vi "OFDM TX - Simulated (No HW).vi"() -> ()   [LabVIEW 2012]
uses:
  <vilib>/addons/Modulation/Analog/controls/Complex Data Waveform.ctl
  <vilib>/addons/Modulation/Digital/General/MT Generate Bits (Galois, PN Order).vi
  <vilib>/addons/Modulation/Digital/General/MT Map Bits to QAM Symbols.vi
  <vilib>/Analysis/2dsp.llb/Inverse Complex FFT.vi
  <vilib>/Analysis/NI_AALPro.lvlib
  <vilib>/addons/Modulation/niDMT.lvlib
  <vilib>/addons/Modulation/niAMT.lvlib
panel:
  out "x*y":cdb[](array[numeric]) format="%#_3g"
  out "Phase":dbl[](graph)
  out "FFT(x)":dbl[](graph)
  in  "Tab Control":T1(tab)=enum."Simulated IQ Impariments"
  in  "IQ rate":dbl=5000000.0 format="%#_6p"
  in  "stop":bool
  out "Outgoing size":i32=1600
  in  "Number of Bits":i32=1250
  in  "error in (no error)":errorcluster
  out "error out":errorcluster
  in  "IQ gain imbalance (dB)":dbl
  in  "frequency offset (Hz)":dbl=250.0
  in  "quadrature skew (deg)":dbl=1.0
  in  "Sample Offset":i32=4
  out "Outgoing Constellation":cdb[](graph)
  # "OFDM Transmitter - Simulated"
  # "Choose offset (0 - 9)"
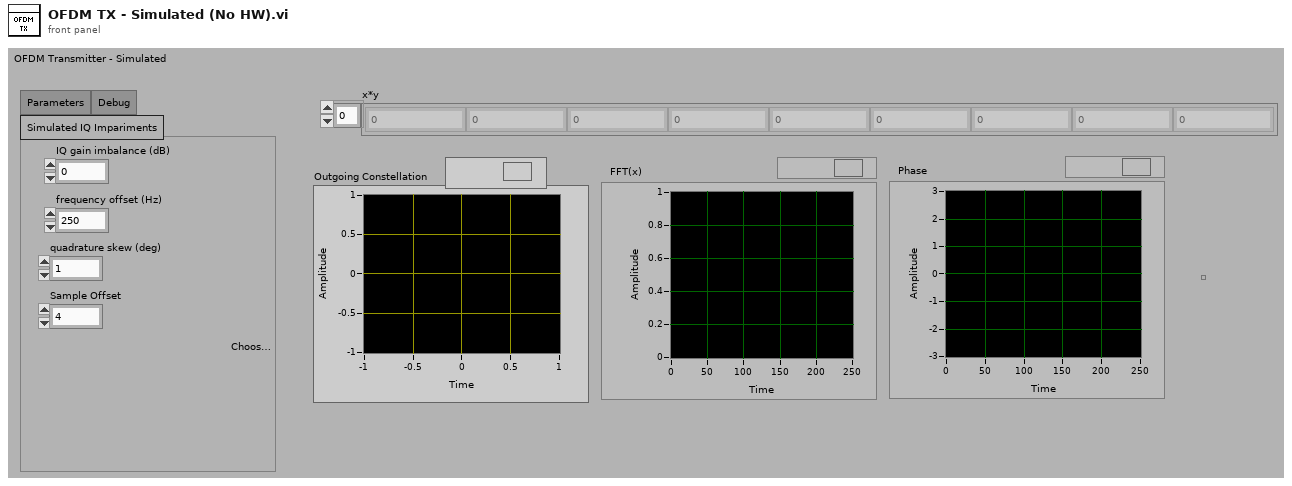
[diagram p1: front panel]
types:
  T1 = enum32{"Parameters", "Debug", "Simulated IQ Impariments"}
  T2 = cluster{"IQ Data":cdb[], "Original Bitstream":i8[]}
  T3 = typedef "niAMT.lvlib/Complex Data Waveform.ctl" = cluster{"t0":dbl, "dt":dbl, "Y":cdb[]}
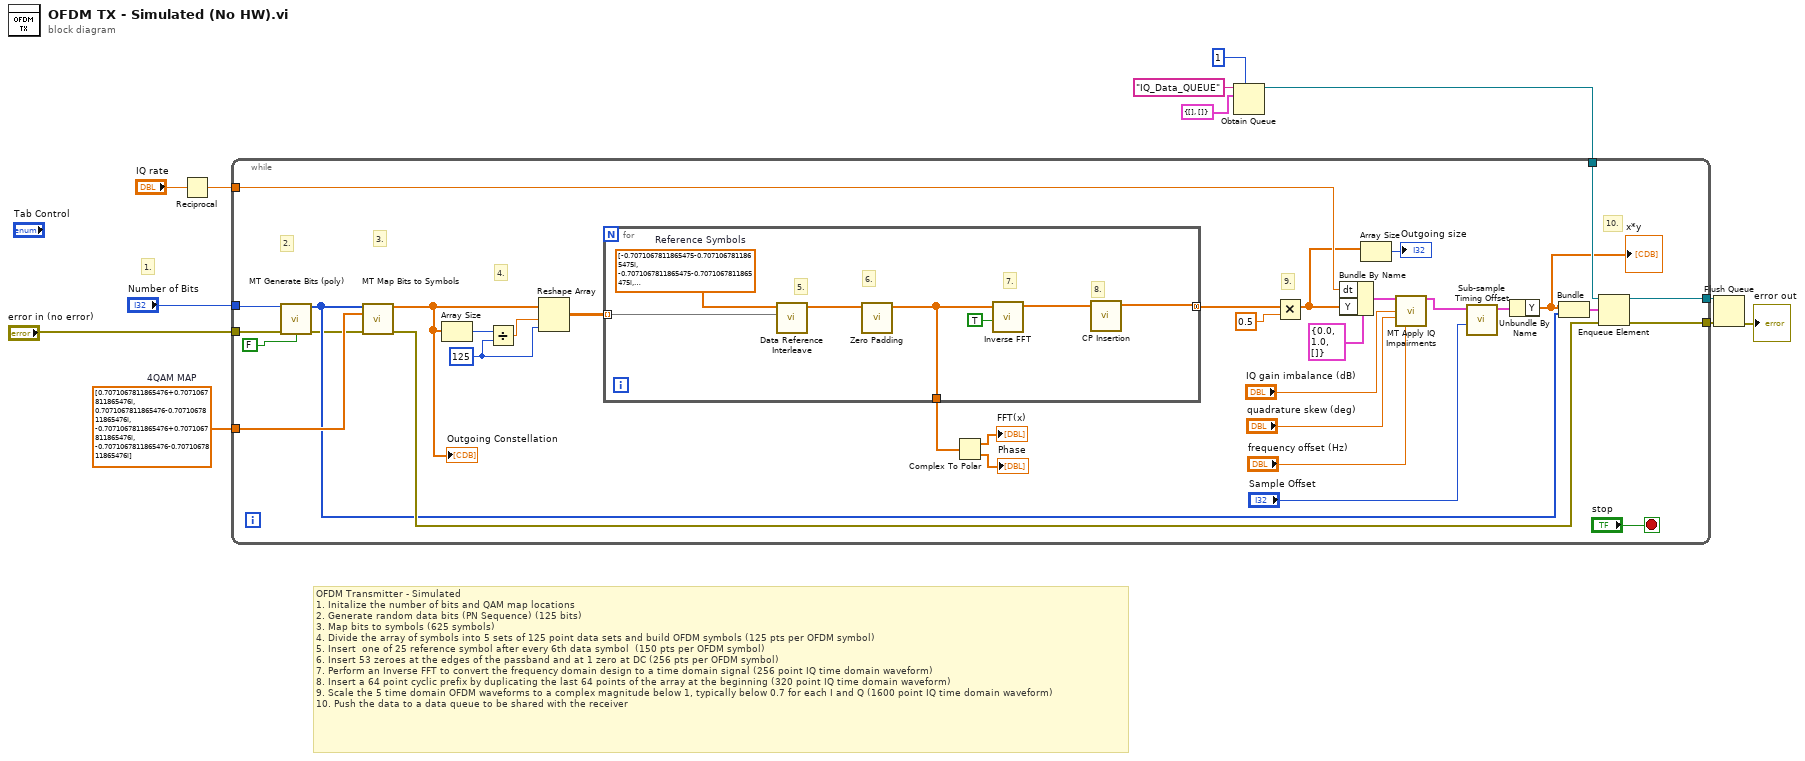
[diagram p0: block diagram]
diagram:
  w12 = cdb[] [0.7071067811865476+0.7071067811865476i, 0.7071067811865476-0.7071067811865476i, -0.7071067811865476+0.7071067811865476i, -0.7071067811865476-0.7071067811865476i]  # 4QAM MAP
  # "1."
  # "OFDM Transmitter - Simulated\n1. Initalize the number of bits and QAM map locations\n2. Generate random data bits (PN Sequence) (125 bits)\n3. Map bits to symbols (625 symbols)\n4. Divide the array of symbols into 5 sets of 125 point data sets and build OFDM symbols (125 pts per OFDM symbol)\n5. Insert  one of 25 reference symbol after every 6th data symbol  (150 pts per OFDM symbol)\n6. Insert 53 zeroes at the edges of the passband and at 1 zero at DC (256 pts per OFDM symbol)\n7. Perform an Inverse FFT to convert the frequency domain design to a time domain signal (256 point IQ time domain waveform)\n8. Insert a 64 point cyclic prefix by duplicating the last 64 points of the array at the beginning (320 point IQ time domain waveform)\n9. Scale the 5 time domain OFDM waveforms to a complex magnitude below 1, typically below 0.7 for each I and Q (1600 point IQ time domain waveform)\n10. Push the data to a data queue to be shared with the receiver"
  n1 = Reciprocal(x="IQ rate") -> (1/x=w3:dbl)
  n2 = Obtain Queue(max queue size (-1, unlimited)=1, name (unnamed)="IQ_Data_QUEUE", element data type=T2 {"IQ Data"=[], "Original Bitstream"=[]} ("output cluster")) -> (queue out=w9:refnum<queue>)  [unwired: 2 in, 2 out]
  n3 = while {
    tunnel: "Number of Bits" -> [w42]
    tunnel: w12 -> [w37]
    tunnel: w9 -> [w31]
    tunnel: [w29] -> w7
    tunnel: [w28] -> w6
    tunnel: w3 -> [w23]
    tunnel: "error in (no error)" -> [w21]
    stop <- "stop" stop-if-true
    w35 = 125 ("y")
    # "10."
    # "9."
    # "4."
    # "3."
    # "2."
    n4 = call-poly <vilib>:"MT Generate Bits (poly).vi"("total bits (128)"=w42, "error in (no error)"=w21, "reset? (T)"=FALSE) -> ("output bit stream"=w15:i8[], "error out"=w13:errorcluster)  [unwired: 10 in, 1 out]
    n5 = call-poly <vilib>:"MT Map Bits to Symbols.vi"("input bit stream"=w15, "symbol map"=w37, "error in (no error)"=w13) -> ("symbols"=w45:cdb[], "error out"=w30:errorcluster)  [unwired: 11 in]
    "Outgoing Constellation" <- w45
    n6 = Array Size(array=w45) -> (size(s)=w44:i32)
    n7 = Divide(x=w44, y=w35) -> (x/y=w43:dbl)
    n8 = Reshape Array(w45, w43, w35) -> (w34:cdb[][])
    n9 = for {
      tunnel: w34 -> [w48] mode=indexing
      tunnel: [w49] -> w32 mode=concatenating
      tunnel: [w51] -> w41
      w47 = cdb[] [-0.7071067811865475-0.7071067811865475i, -0.7071067811865475-0.7071067811865475i, -0.7071067811865475-0.7071067811865475i, 0.7071067811865475-0.7071067811865475i, 0.7071067811865475-0.7071067811865475i, 0.7071067811865475+0.7071067811865475i, 0.7071067811865475-0.7071067811865475i, -0.7071067811865475-0.7071067811865475i, 0.7071067811865475+0.7071067811865475i, -0.7071067811865475+0.7071067811865475i, -0.7071067811865475-0.7071067811865475i, -0.7071067811865475+0.7071067811865475i, -0.7071067811865475+0.7071067811865475i, 0.7071067811865475-0.7071067811865475i, -0.7071067811865475+0.7071067811865475i, -0.7071067811865475+0.7071067811865475i, 0.7071067811865475-0.7071067811865475i, -0.7071067811865475+0.7071067811865475i, -0.7071067811865475-0.7071067811865475i, 0.7071067811865475-0.7071067811865475i, 0.7071067811865475+0.7071067811865475i, -0.7071067811865475-0.7071067811865475i, -0.7071067811865475-0.7071067811865475i, 0.7071067811865475-0.7071067811865475i, -0.7071067811865475-0.7071067811865475i, 0.7071067811865475-0.7071067811865475i, 0.7071067811865475-0.7071067811865475i, 0.7071067811865475+0.7071067811865475i, 0.7071067811865475+0.7071067811865475i, -0.7071067811865475-0.7071067811865475i, -0.7071067811865475+0.7071067811865475i, -0.7071067811865475+0.7071067811865475i, 0.7071067811865475-0.7071067811865475i, -0.7071067811865475-0.7071067811865475i, -0.7071067811865475+0.7071067811865475i, -0.7071067811865475-0.7071067811865475i, -0.7071067811865475+0.7071067811865475i, 0.7071067811865475-0.7071067811865475i, 0.7071067811865475+0.7071067811865475i, 0.7071067811865475+0.7071067811865475i, 0.7071067811865475-0.7071067811865475i, -0.7071067811865475-0.7071067811865475i, -0.7071067811865475+0.7071067811865475i, -0.7071067811865475+0.7071067811865475i, -0.7071067811865475-0.7071067811865475i, -0.7071067811865475-0.7071067811865475i, -0.7071067811865475+0.7071067811865475i, -0.7071067811865475+0.7071067811865475i, -0.7071067811865475+0.7071067811865475i, -0.7071067811865475+0.7071067811865475i]  # Reference Symbols
      # "8."
      # "7."
      # "6."
      # "5."
      n10 = call <userlib>:"Data Reference Interleave.vi"("Data Symbols"=w48, "Reference Symbols"=w47) -> ("Interleaved Output"=w50:cdb[])  [unwired: 9 in]
      n11 = call <userlib>:"Zero Padding.vi"("Array in"=w50) -> ("Array out"=w51:cdb[])  [unwired: 10 in]
      n12 = call-poly <vilib>:"Inverse FFT.vi"("shift?"=TRUE, "FFT {X}"=w51) -> ("X"=w52:cdb[])  [unwired: 8 in, 1 out]
      n13 = call <userlib>:"CP Insertion.vi"("Input"=w52) -> ("Output with CP"=w49:cdb[])  [unwired: 10 in]
    }
    n14 = Complex To Polar(r * e^(i*theta)=w41) -> (r=→"FFT(x)":dbl[], theta=→"Phase":dbl[])
    n15 = Multiply(x=w32, y=0.5 ("value")) -> (x*y=w17:cdb[])
    n16 = Bundle By Name(cluster=T3 {"t0"=0.0, "dt"=1.0, "Y"=[]} ("input complex waveform"), "dt"=w23, "Y"=w17) -> (w27:T3)
    n17 = Array Size(array=w17) -> (size(s)=→"Outgoing size":i32)
    n18 = call <vilib>:"MT Apply IQ Impairments.vi"("input complex waveform"=w27, "IQ gain imbalance (dB)"="IQ gain imbalance (dB)", "quadrature skew (deg)"="quadrature skew (deg)", "frequency offset (Hz)"="frequency offset (Hz)") -> ("output complex waveform"=w19:T3)  [unwired: 10 in, 1 out]
    n19 = call <userlib>:"Sub-sample Timing Offset.vi"("Sample Offset"="Sample Offset", "output complex waveform in"=w19) -> ("output complex waveform out"=w20:T3)  [unwired: 9 in]
    n20 = Unbundle By Name(w20) -> ("Y"=w16:cdb[])
    "x*y" <- w16
    n21 = Bundle("Y"=w16, "output bit stream"=w15) -> (w14:cluster{"Y":cdb[], "output bit stream":i8[]})  [unwired: 1 in]
    n22 = Enqueue Element(queue=w31, element=w14, error in (no error)=w30) -> (queue out=w29:refnum<queue>, error out=w28:errorcluster)  [unwired: 1 in, 1 out]
  }
  n23 = Flush Queue(queue=w7, error in (no error)=w6) -> (error out=→"error out":errorcluster)  [unwired: 2 out]
